vi "True Color To Indexed Color Image.vi"(8 "error in (no error)":errorcluster, 9 "Dither (None)":T1, 10 "Depth (8)":i32=8, 11 "True Color Image":T2) -> (0 "error out":errorcluster, 3 "Indexed Image":T2)   [LabVIEW 2020, in "G-Image.lvlib"]
doc: "Convert a 24-bit or 32-bit image to an indexed color image.\n\nDepth defines the number of colors in the indexed image:\n8-bit => 256 colors\n7-bit =>128 colors\n...\n\nThe resulting indexed image will always be 8-bit"
uses:
  G-Image.lvlib
  <vilib>/picture/picture.llb/imagedata.ctl
  Image IO/Controls/Dither Type.ctl
  <vilib>/Utility/error.llb/Error Cluster From Error Code.vi
  lib/g_image_32.dll
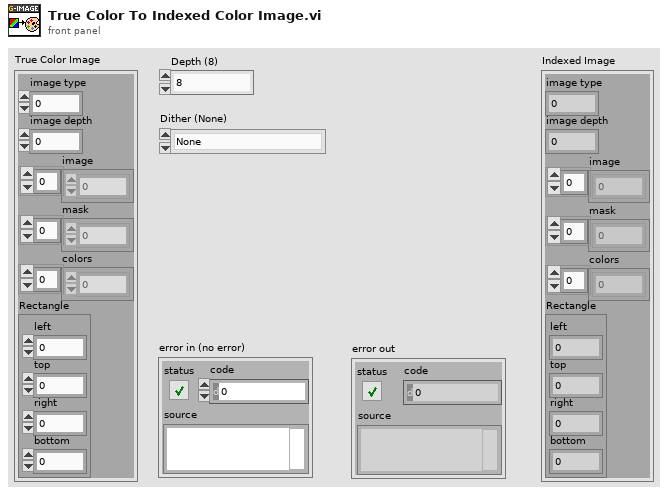
[diagram p1: front panel]
types:
  T1 = typedef "G-Image.lvlib/Dither Type.ctl" = enum32{"None", "Floyd-Steinberg"}
  T2 = typedef "imagedata.ctl" = cluster{"image type":i32, "image depth":i32, "image":u8[], "mask":u8[], "colors":u32[], "Rectangle":cluster{"left":i16, "top":i16, "right":i16, "bottom":i16}}
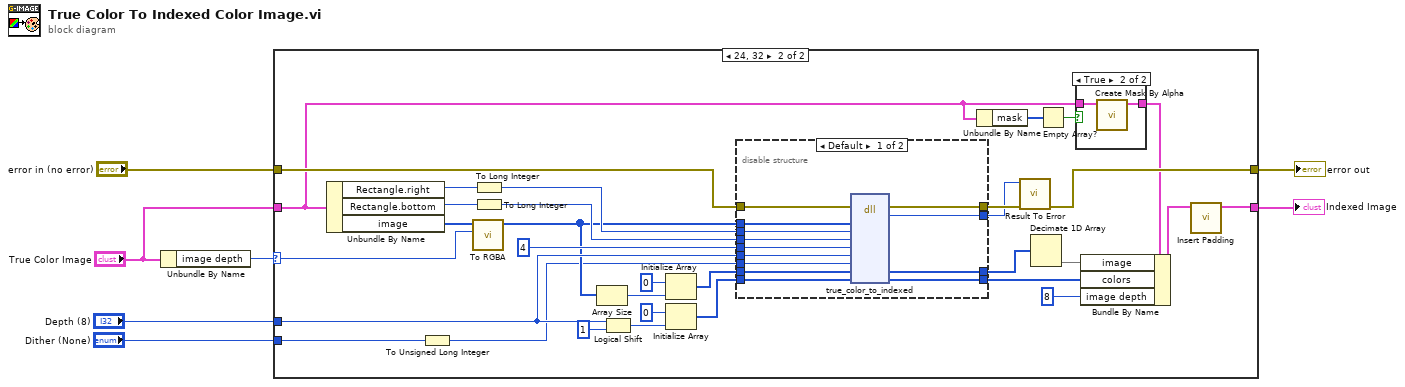
[diagram p0: block diagram]
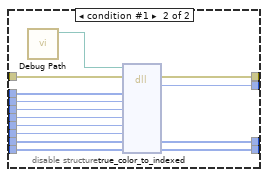
[diagram p4: hidden frame]
diagram:
  n1 = Unbundle By Name("True Color Image") -> ("image depth"=w7:i32)
  n2 = case shown="24, 32" w7 {
    selector: w7 -> [_ w41]
    tunnel: [w9 w14] -> w5
    tunnel: "True Color Image" -> [w9 w12]
    tunnel: "Depth (8)" -> [_ w25]
    tunnel: "Dither (None)" -> [_ w40]
    tunnel: "error in (no error)" -> [w8 w26]
    tunnel: [w8 w23] -> w1
    frame Default {
    }
    frame 24, 32 {
      n3 = Unbundle By Name(w12) -> ("Rectangle.right"=w39:i16, "Rectangle.bottom"=w38:i16, "image"=w31:u8[])
      n4 = To Unsigned Long Integer(number=w40) -> (unsigned 32bit integer=w17:u32)
      n5 = call "To RGBA.vi"("Depth"=w41, "Image Data"=w31) -> ("RGBA"=w21:u8[])  [unwired: 9 in]
      n6 = To Long Integer(number=w39) -> (32bit integer=w29:i32)
      n7 = To Long Integer(number=w38) -> (32bit integer=w30:i32)
      n8 = Array Size(array=w21) -> (size(s)=w20:i32)
      n9 = Logical Shift(y=w25, x=u32 1) -> (x << y=w34:u32)
      n10 = Initialize Array(u8 0 ("element"), w20) -> (w28:u8[])
      n11 = Initialize Array(u32 0 ("element"), w34) -> (w27:u32[])
      n12 = disable-structure shown="Default" {
        disable-tunnel: [w57 w70] -> w33
        disable-tunnel: w26 -> [w56 w68]
        disable-tunnel: [w55 w69] -> w32
        disable-tunnel: w21 -> [w54 w67]
        disable-tunnel: w29 -> [w53 w66]
        disable-tunnel: w30 -> [w52 w65]
        disable-tunnel: 4 ("Channels") -> [w51 w64]
        disable-tunnel: w25 -> [w46 w63]
        disable-tunnel: w17 -> [w45 w62]
        disable-tunnel: w28 -> [w50 w61]
        disable-tunnel: [w49 w58] -> w19
        disable-tunnel: w27 -> [w48 w60]
        disable-tunnel: [w47 w59] -> w24
        frame condition #0 (active) {
          n13 = dll-call lib="C:/github/dataflowg/g-image/src/LabVIEW/G-Image/lib/g_image_*.*" fn="true_color_to_indexed"(error in=w56, "image_data_in"=w54, "width_in"=w53, "height_in"=w52, "channels_in"=w51, "depth"=w46, "dither"=w45, "image_data_out"=w50, "colors_out"=w48) -> (error out=w57:errorcluster, "result"=w55:i32, "image_data_out"=w49:u8[], "colors_out"=w47:u32[])  [unwired: 8 in, 1 out]
        }
        frame condition #1 {
          n14 = call "Debug Path.vi"() -> ("Debug Path"=w71:path)  [unwired: 11 in]
          n15 = dll-call lib="?" fn="true_color_to_indexed"(path in=w71, error in=w68, "image_data_in"=w67, "width_in"=w66, "height_in"=w65, "channels_in"=w64, "depth"=w63, "dither"=w62, "image_data_out"=w61, "colors_out"=w60) -> (error out=w70:errorcluster, "result"=w69:i32, "image_data_out"=w58:u8[], "colors_out"=w59:u32[])  [unwired: 7 in, 1 out]
        }
      }
      n16 = Unbundle By Name(w12) -> ("mask"=w11:u8[])
      n17 = call "Result To Error.vi"("error in (no error)"=w33, "Result Code"=w32) -> ("error out"=w23:errorcluster)  [unwired: 9 in]
      n18 = Decimate 1D Array(w19) -> (w16:u8[])  [unwired: 3 out]
      n19 = Empty Array?(array=w11) -> (empty?=w10:bool)
      n20 = case shown="True" w10 {
        tunnel: [w42 w44] -> w13
        tunnel: w12 -> [w42 w43]
        frame False {
        }
        frame True {
          n21 = call <vilib>:"Create Mask By Alpha.vi"("image data"=w43) -> ("masked image data"=w44:T2)  [unwired: 10 in]
        }
      }
      n22 = Bundle By Name(cluster=w13, "image"=w16, "colors"=w24, "image depth"=8) -> (w15:T2)
      n23 = call "Insert Padding.vi"("Image"=w15) -> ("Image Out"=w14:T2)  [unwired: 9 in, 1 out]
    }
  }
  "error out" <- w1
  "Indexed Image" <- w5
